vi "Possible Coords after Step.vi"(10 "Steps":i32, 11 "Proto in":refnum<class "Proto.lvclass">) -> (3 "Array":cluster{"Row":i32, "Col":i32}[](array[cluster]))   [LabVIEW 2021, in "Proto.lvclass"]
uses:
  Proto.lvclass
  Proto.lvclass/Proto.ctl
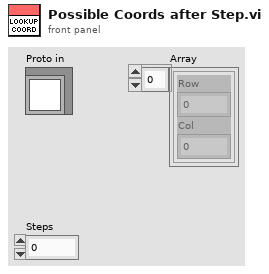
[diagram p1: front panel]
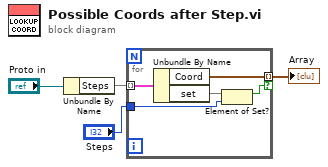
[diagram p0: block diagram]
diagram:
  n1 = Unbundle By Name("Proto in") -> ("Steps"=w2:map{cluster{"Row":i32, "Col":i32}, set{i32}})
  n2 = for {
    tunnel: w2 -> [w9] mode=indexing
    tunnel: "Steps" -> [w7]
    tunnel: [w6] -> w3 mode=indexing if=w5
    n3 = Unbundle By Name(w9) -> ("Coord"=w6:cluster{"Row":i32, "Col":i32}, "set"=w8:set{i32})
    n4 = Element of Set?(10:w7, 11:w8) -> (3:w5:bool)
  }
  "Array" <- w3
